vi "Check_Measurement_Setups.vi"(0 "Measurement Setup String":string) -> (1 "Measurement Setup String Out":string, 2 "Error Comments":string)   [LabVIEW 2010]
uses:
  Globals/Constants_global.vi
  Globals/Trav_pos_global.vi
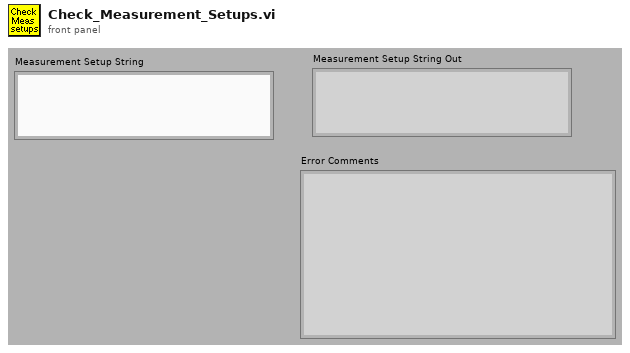
[diagram p1: front panel]
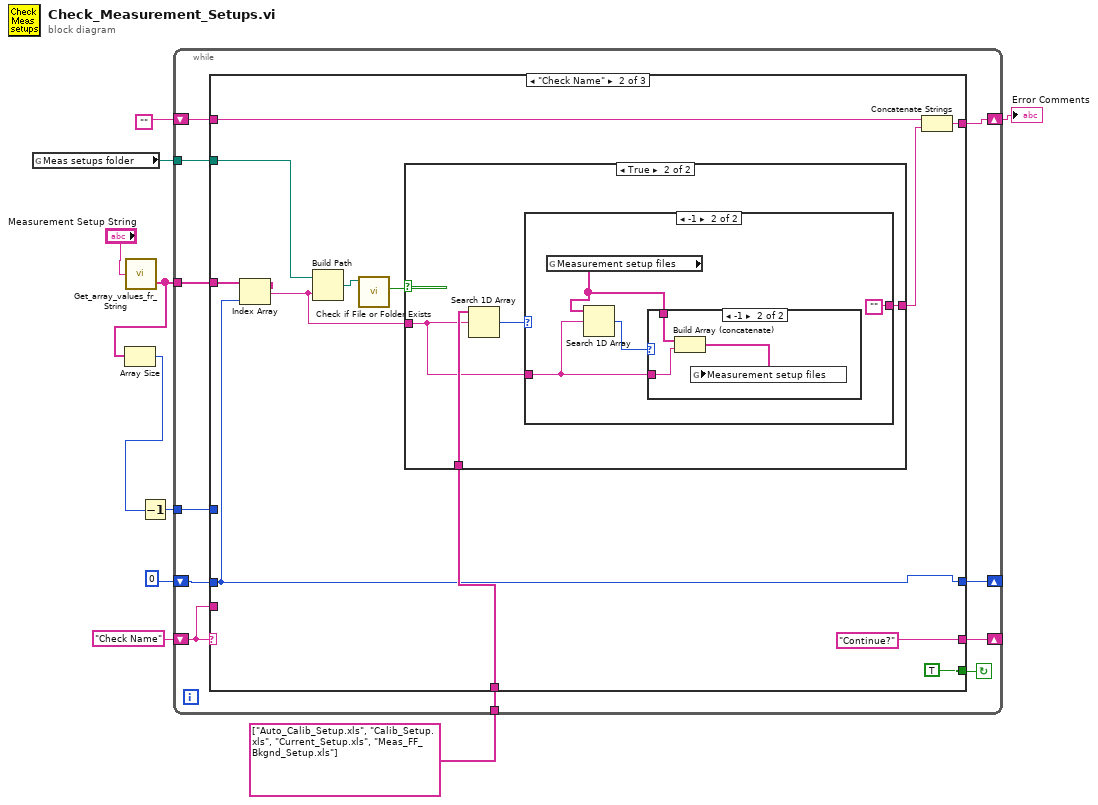
[diagram p0: block diagram]
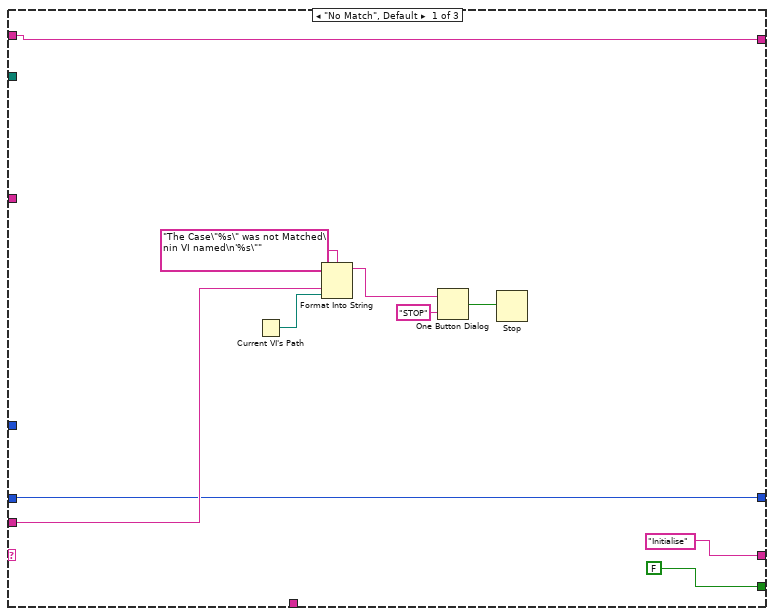
[diagram p2: hidden frame]
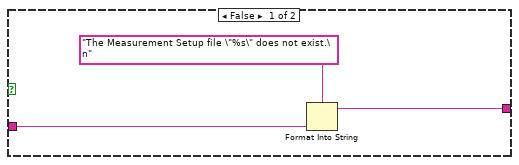
[diagram p3: hidden frame]
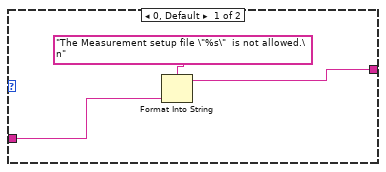
[diagram p4: hidden frame]
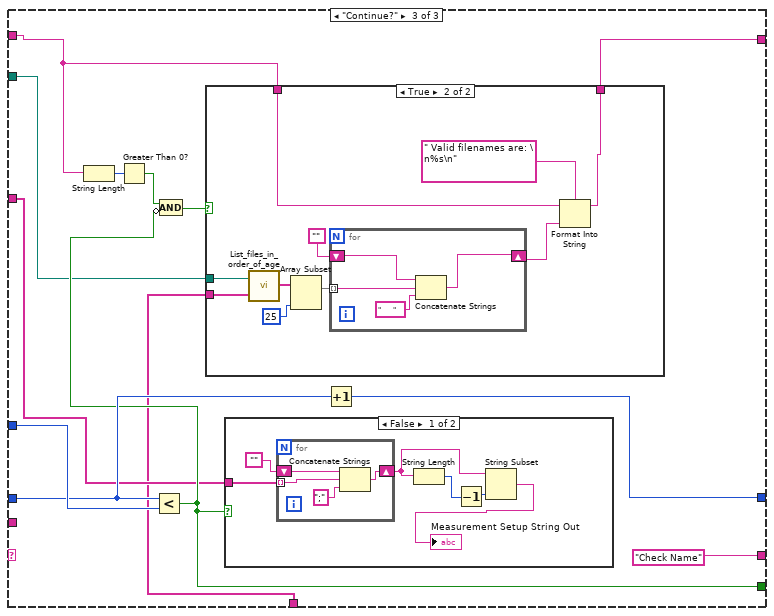
[diagram p6: hidden frame]
diagram:
  n1 = global read "Constants_global.vi" "Meas setups folder"() -> (w7:path)
  n2 = call "Get_array_values_fr_String.vi"("String Value"="Measurement Setup String") -> ("String array"=w6:string[])  [unwired: 1 out]
  n3 = Array Size(array=w6) -> (size(s)=w5:i32)
  n4 = Decrement(x=w5) -> (x-1=w4:i32)
  n5 = while {
    shift-left: "Check Name" -> [w19]
    shift-right: [w20] -> _
    shift-right: [w14] -> _
    shift-left: 0 -> [w18]
    tunnel: w6 -> [w17]
    tunnel: w7 -> [w16]
    tunnel: w4 -> [w15]
    shift-right: [w13] -> w1
    shift-left: "" -> [w12]
    tunnel: string[] ["Auto_Calib_Setup.xls", "Calib_Setup.xls", "Current_Setup.xls", "Meas_FF_Bkgnd_Setup.xls"] ("file names") -> [w11]
    stop <- w21 continue-if-true
    n6 = case shown="\"Check Name\"" w19 {
      tunnel: [FALSE TRUE w64] -> w21
      tunnel: ["Initialise" "Continue?" "Check Name"] -> w20
      tunnel: w19 -> [w26 _ _]
      tunnel: w18 -> [w23 w32 w72]
      tunnel: w17 -> [_ w43 w63]
      tunnel: w16 -> [_ w42 w61]
      tunnel: w15 -> [_ _ w73]
      tunnel: [w23 w32 w71] -> w14
      tunnel: [w22 w38 w65] -> w13
      tunnel: w12 -> [w22 w36 w66]
      tunnel: w11 -> [_ w33 w62]
      frame "No Match", Default {
        n7 = Current VI's Path() -> (path=w25:path)
        n8 = Format Into String(format string="The Case\"%s\" was not Matched\nin VI named\n'%s\"" ("Format String"), w26, w25) -> (resulting string=w29:string)  [unwired: 2 in, 1 out]
        n9 = One Button Dialog(message=w29, button name ("OK")="STOP") -> (true=w27:bool)
        n10 = Stop(stop? (T)=w27) -> ()
      }
      frame "Check Name" {
        n11 = Index Array(array=w43, index=w32) -> (element=w39:string)
        n12 = Build Path(base path=w42, name or relative path=w39) -> (appended path=w40:path)
        n13 = call <vilib>:"Check if File or Folder Exists.vi"("path"=w40) -> ("file or folder exists?"=w41:bool)  [unwired: 1 in, 9 out]
        n14 = case shown="True" w41 {
          tunnel: w39 -> [w45 w47]
          tunnel: [w44 w48] -> w37
          tunnel: w33 -> [_ w50]
          frame False {
            n15 = Format Into String(format string="The Measurement Setup file \"%s\" does not exist.\n" ("Format String"), w45) -> (resulting string=w44:string)  [unwired: 2 in, 1 out]
          }
          frame True {
            n16 = Search 1D Array(1D array=w50, element=w47) -> (index of element=w49:i32)  [unwired: 1 out]
            n17 = case shown="-1" w49 {
              tunnel: [w52 ""] -> w48
              tunnel: w47 -> [w51 w55]
              frame 0, Default {
                n18 = Format Into String(format string="The Measurement setup file \"%s\"  is not allowed.\n" ("f"), w51) -> (resulting string=w52:string)  [unwired: 2 in, 1 out]
              }
              frame -1 {
                n19 = global read "Trav_pos_global.vi" "Measurement setup files"() -> (w56:string[])
                n20 = Search 1D Array(1D array=w56, element=w55) -> (index of element=w57:i32)  [unwired: 1 out]
                n21 = case shown="-1" w57 {
                  tunnel: w56 -> [_ w60]
                  tunnel: w55 -> [_ w59]
                  frame 0, Default {
                  }
                  frame -1 {
                    n22 = Build Array (concatenate)(w60, w59) -> (w58:string[])
                    n23 = global write "Trav_pos_global.vi" "Measurement setup files"(w58) -> ()
                  }
                }
              }
            }
          }
        }
        n24 = Concatenate Strings(w36, w37) -> (w38:string)
      }
      frame "Continue?" {
        n25 = String Length(string=w66) -> (length=w69:i32)
        n26 = Greater Than 0?(x=w69) -> (x > 0?=w68:bool)
        n27 = Less?(x=w72, y=w73) -> (x < y?=w64:bool)
        n28 = Compound Arithmetic op=AND(w68, invert w64) -> (w67:bool)
        n29 = case shown="True" w67 {
          tunnel: w66 -> [w84 w88]
          tunnel: [w84 w87] -> w65
          tunnel: w62 -> [_ w86]
          tunnel: w61 -> [_ w85]
          frame False {
          }
          frame True {
            n30 = call "List_files_in_order_of_age.vi"("Files to Hide"=w86, "Folder"=w85) -> ("file names"=w90:string[])
            n31 = Array Subset(array=w90, length=25 ("Array Length")) -> (w92:string[])  [unwired: 1 in]
            n32 = for {
              shift-right: [w97] -> w94
              shift-left: "" -> [w98]
              tunnel: w92 -> [w96] mode=indexing
              n33 = Concatenate Strings(w98, w96, "      " ("Substring")) -> (w97:string)
            }
            n34 = Format Into String(format string=" Valid filenames are: \n%s\n" ("Format String"), initial string=w88, w94) -> (resulting string=w87:string)  [unwired: 1 in, 1 out]
          }
        }
        n35 = case shown="False" w64 {
          tunnel: w63 -> [w79 _]
          frame False {
            n36 = for {
              shift-right: [w80] -> w76
              shift-left: "" -> [w83]
              tunnel: w79 -> [w82] mode=indexing
              n37 = Concatenate Strings(w83, w82, ";") -> (w80:string)
            }
            n38 = String Length(string=w76) -> (length=w77:i32)
            n39 = Decrement(x=w77) -> (x-1=w75:i32)
            n40 = String Subset(string=w76, length (rest)=w75) -> (substring=→"Measurement Setup String Out":string)  [unwired: 1 out]
          }
          frame True {
          }
        }
        n41 = Increment(x=w72) -> (x+1=w71:i32)
      }
    }
  }
  "Error Comments" <- w1
